vi "find-project-application-by-name.vi"(0 "Application Reference in":refnum<vi>, 5 "Project Name":string, 11 "error in (no error)":errorcluster) -> (4 "Application Reference out":refnum<vi>, 6 "Project Application Ref":refnum<vi>, 15 "error out":errorcluster)   [LabVIEW 2016]
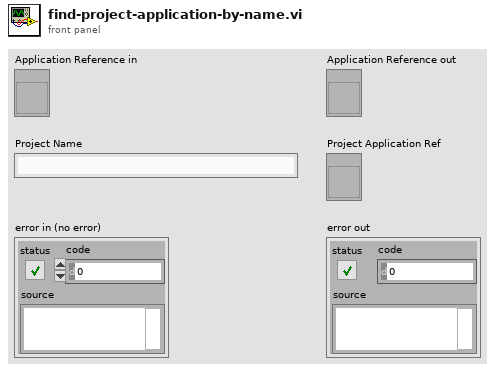
[diagram p1: front panel]
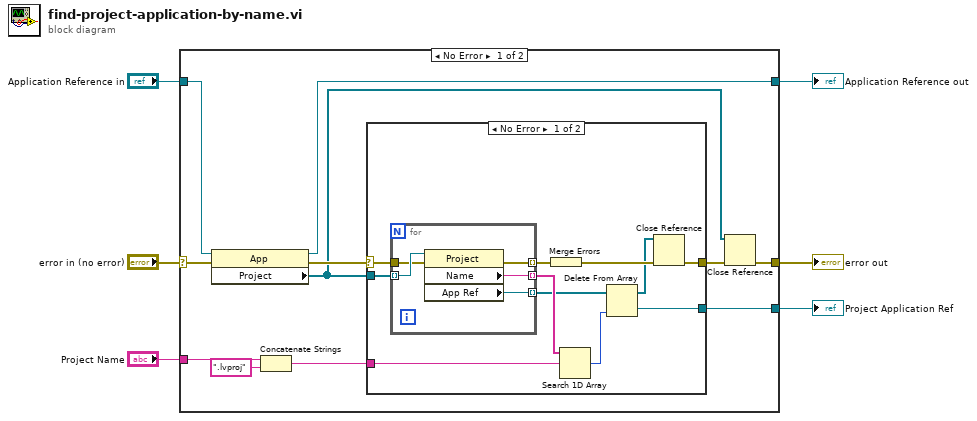
[diagram p0: block diagram]
diagram:
  n1 = case shown="No Error" "error in (no error)" {
    selector: "error in (no error)" -> [w17 w36]
    tunnel: "Application Reference in" -> [w16 w35]
    tunnel: [w15 w35] -> w4
    tunnel: [w12 w36] -> w3
    tunnel: "Project Name" -> [w10 _]
    tunnel: [w9 _] -> w1
    frame No Error {
      n2 = property class="App"(reference=w16, error in=w17) -> (reference out=w15:refnum<vi>, error out=w14:errorcluster, "Project"=w11:refnum<vi>[])
      n3 = Concatenate Strings(w10, ".lvproj" ("string")) -> (w8:string)
      n4 = case shown="No Error" w14 {
        selector: w14 -> [w27 w34]
        tunnel: w11 -> [w28 _]
        tunnel: [w20 w34] -> w13
        tunnel: w8 -> [w25 _]
        tunnel: [w18 _] -> w9
        frame No Error {
          n5 = for {
            tunnel: w28 -> [w33] mode=indexing
            tunnel: w27 -> [w32]
            tunnel: [w31] -> w24 mode=indexing
            tunnel: [w30] -> w26 mode=indexing
            tunnel: [w29] -> w23 mode=indexing
            n6 = property class="Project"(reference=w33, error in=w32) -> (error out=w29:errorcluster, "Name"=w30:string, "App Ref"=w31:refnum<vi>)  [unwired: 1 out]
          }
          n7 = Merge Errors(w23) -> (w22:errorcluster)
          n8 = Search 1D Array(1D array=w26, element=w25) -> (index of element=w21:i32)  [unwired: 1 in]
          n9 = Delete From Array(array=w24, index=w21) -> (deleted portion=w18:refnum<vi>, array with subset deleted=w19:refnum<vi>[])  [unwired: 1 in]
          n10 = Close Reference(reference=w19, error in (no error)=w22) -> (error out=w20:errorcluster)
        }
        frame Error {
        }
      }
      n11 = Close Reference(reference=w11, error in (no error)=w13) -> (error out=w12:errorcluster)
    }
    frame Error {
    }
  }
  "Application Reference out" <- w4
  "error out" <- w3
  "Project Application Ref" <- w1
